vi "Read AttrName.vi"(11 "Attribute in":refnum<class "Attribute.lvclass">) -> (2 "Attribute Name":string, 3 "Attribute out":refnum<class "Attribute.lvclass">, 5 "unnamed":bool)   [LabVIEW 2021, in "smo.lvlib" / "Attribute.lvclass"]
uses:
  Attribute.lvclass
  Attribute.lvclass/Attribute.ctl
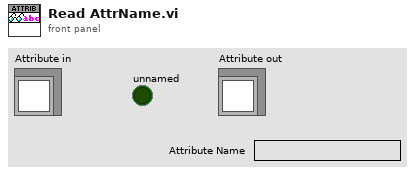
[diagram p1: front panel]
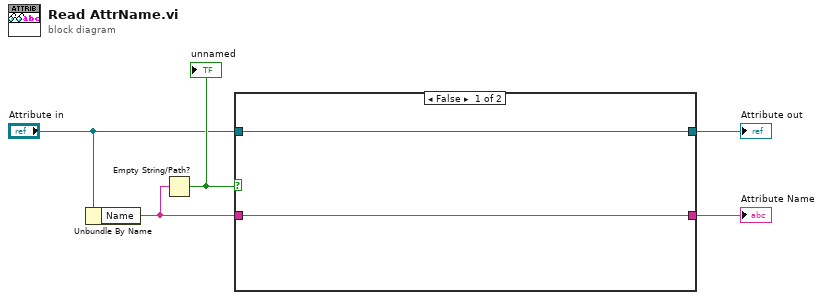
[diagram p0: block diagram]
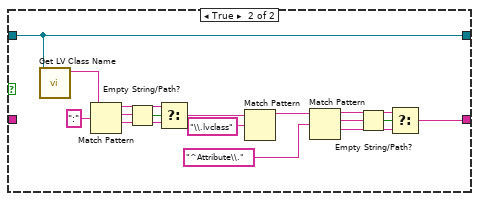
[diagram p2: hidden frame]
diagram:
  n1 = Unbundle By Name("Attribute in") -> ("Name"=w1:string)
  n2 = Empty String/Path?(string/path=w1) -> (empty?=w5:bool)
  "unnamed" <- w5
  n3 = case shown="False" w5 {
    tunnel: "Attribute in" -> [w7 w23]
    tunnel: [w7 w23] -> w4
    tunnel: [w6 w8] -> w2
    tunnel: w1 -> [w6 _]
    frame False {
    }
    frame True {
      n4 = call <vilib>:"Get LV Class Name.vi"("object"=w23) -> ("class name"=w22:string)  [unwired: 9 in, 1 out]
      n5 = Match Pattern(string=w22, regular expression=":") -> (before substring=w17:string, match substring=w19:string, after substring=w16:string)  [unwired: 1 in, 1 out]
      n6 = Empty String/Path?(string/path=w19) -> (empty?=w18:bool)
      n7 = Select(t=w17, s=w18, f=w16) -> (s? t:f=w15:string)
      n8 = Match Pattern(string=w15, regular expression="\\.lvclass") -> (before substring=w9:string)  [unwired: 1 in, 3 out]
      n9 = Match Pattern(string=w9, regular expression="^Attribute\\.") -> (before substring=w11:string, match substring=w12:string, after substring=w10:string)  [unwired: 1 in, 1 out]
      n10 = Empty String/Path?(string/path=w12) -> (empty?=w13:bool)
      n11 = Select(t=w11, s=w13, f=w10) -> (s? t:f=w8:string)
    }
  }
  "Attribute out" <- w4
  "Attribute Name" <- w2
